vi "SDCP Receiver and Transmitter - Limit Parameter Values.vi"(3 "error in (no error)":errorcluster, 4 "Parameter descriptor in":T1, 5 "Parameter value in":string) -> (0 "error out":errorcluster, 2 "Parameter value out":string)   [LabVIEW 2020]
uses:
  Typedefs/SDCP - SMF parameter descriptors.ctl
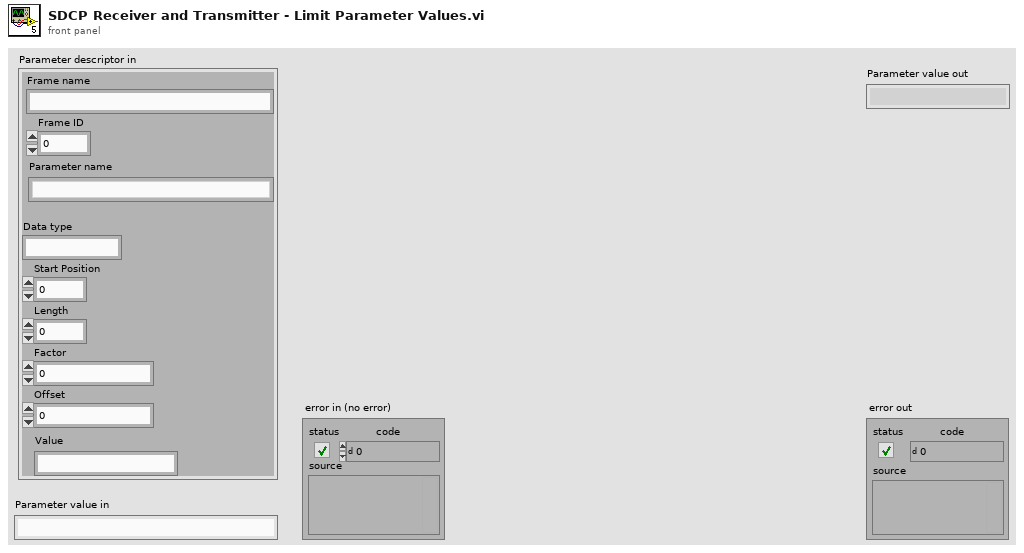
[diagram p1: front panel]
types:
  T1 = typedef "SDCP - SMF parameter descriptors.ctl" = cluster{"Frame name":string, "Frame ID":i32, "Data type":string, "Start Position":i32, "Length":i32, "Factor":dbl, "Offset":dbl, "Parameter name":string, "Value":string}
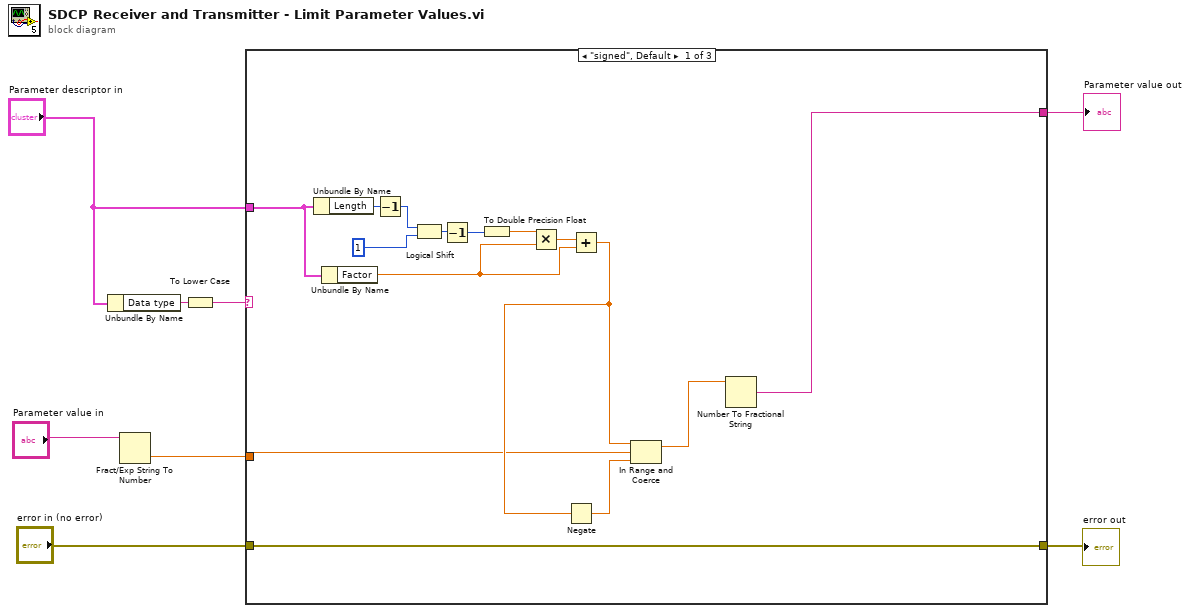
[diagram p0: block diagram]
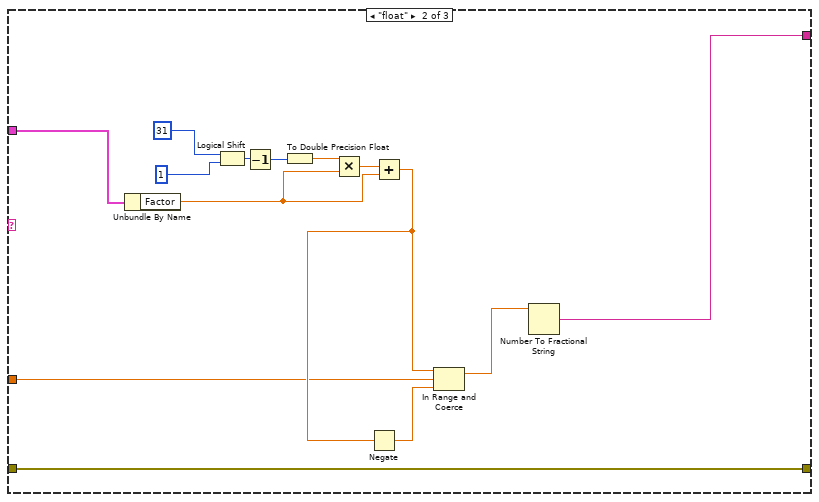
[diagram p2: hidden frame]
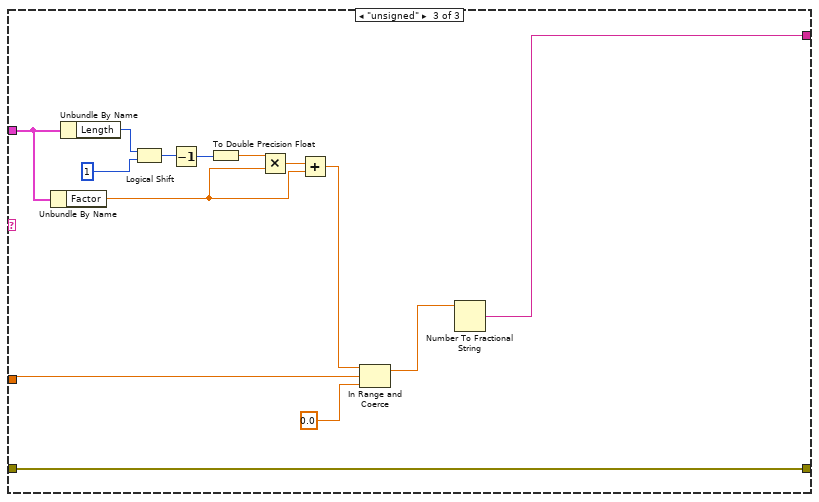
[diagram p3: hidden frame]
diagram:
  n1 = Unbundle By Name("Parameter descriptor in") -> ("Data type"=w2:string)
  n2 = Fract/Exp String To Number(string="Parameter value in") -> (number=w6:dbl)  [unwired: 3 in, 1 out]
  n3 = To Lower Case(string=w2) -> (all lower case string=w1:string)
  n4 = case shown="\"signed\", Default" w1 {
    tunnel: "error in (no error)" -> [w9 w24 w38]
    tunnel: w6 -> [w11 w27 w41]
    tunnel: "Parameter descriptor in" -> [w15 w28 w46]
    tunnel: [w10 w25 w39] -> w4
    tunnel: [w9 w24 w38] -> w3
    frame "signed", Default {
      n5 = Unbundle By Name(w15) -> ("Length"=w22:i32)
      n6 = Unbundle By Name(w15) -> ("Factor"=w17:dbl)
      n7 = Decrement(x=w22) -> (x-1=w14:i32)
      n8 = Logical Shift(y=w14, x=u64 1) -> (x << y=w21:u64)
      n9 = Decrement(x=w21) -> (x-1=w20:u64)
      n10 = To Double Precision Float(number=w20) -> (double precision float=w19:dbl)
      n11 = Multiply(x=w19, y=w17) -> (x*y=w18:dbl)
      n12 = Add(x=w18, y=w17) -> (x+y=w12:dbl)
      n13 = Negate(x=w12) -> (-x=w13:dbl)
      n14 = In Range and Coerce(upper limit=w12, x=w11, lower limit=w13) -> (coerced(x)=w16:dbl)  [unwired: 1 out]
      n15 = Number To Fractional String(number=w16) -> (F-format string=w10:string)  [unwired: 3 in]
    }
    frame "float" {
      n16 = Unbundle By Name(w28) -> ("Factor"=w32:dbl)
      n17 = Logical Shift(y=i16 31, x=u64 1) -> (x << y=w36:u64)
      n18 = Decrement(x=w36) -> (x-1=w35:u64)
      n19 = To Double Precision Float(number=w35) -> (double precision float=w34:dbl)
      n20 = Multiply(x=w34, y=w32) -> (x*y=w33:dbl)
      n21 = Add(x=w33, y=w32) -> (x+y=w29:dbl)
      n22 = Negate(x=w29) -> (-x=w30:dbl)
      n23 = In Range and Coerce(upper limit=w29, x=w27, lower limit=w30) -> (coerced(x)=w31:dbl)  [unwired: 1 out]
      n24 = Number To Fractional String(number=w31) -> (F-format string=w25:string)  [unwired: 3 in]
    }
    frame "unsigned" {
      n25 = Unbundle By Name(w46) -> ("Factor"=w44:dbl)
      n26 = Unbundle By Name(w46) -> ("Length"=w50:i32)
      n27 = Logical Shift(y=w50, x=u64 1) -> (x << y=w49:u64)
      n28 = Decrement(x=w49) -> (x-1=w48:u64)
      n29 = To Double Precision Float(number=w48) -> (double precision float=w47:dbl)
      n30 = Multiply(x=w47, y=w44) -> (x*y=w45:dbl)
      n31 = Add(x=w45, y=w44) -> (x+y=w42:dbl)
      n32 = In Range and Coerce(upper limit=w42, x=w41, lower limit=0.0) -> (coerced(x)=w40:dbl)  [unwired: 1 out]
      n33 = Number To Fractional String(number=w40) -> (F-format string=w39:string)  [unwired: 3 in]
    }
  }
  "error out" <- w3
  "Parameter value out" <- w4
